vi "ax+b(double).vi"(1 "x":dbl, 2 "b":dbl, 3 "a":dbl) -> (0 "y":dbl)   [LabVIEW 2012]
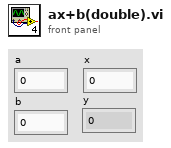
[diagram p1: front panel]
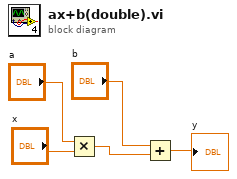
[diagram p0: block diagram]
diagram:
  n1 = Multiply(x="a", y="x") -> (x*y=w3:dbl)
  n2 = Add(x="b", y=w3) -> (x+y=→"y":dbl)
